vi "Conversion Lookup Table Get Conversion Parameter.vi"(8 "error in (no error)":errorcluster, 10 "ID":u32, 11 "Ref in":T2) -> (0 "error out":errorcluster {"code" min=0 max=0}, 1 "Found?":bool, 2 "Parameters":T1, 3 "vi reference":T2)   [LabVIEW 2013, in "J1939.lvlib"]
uses:
  J1939.lvlib
  LUTs/J1939 Conversion Lookup Table Reference.ctl
  LUTs/J1939 Conversion Lookup Table Parameters Cluster.ctl
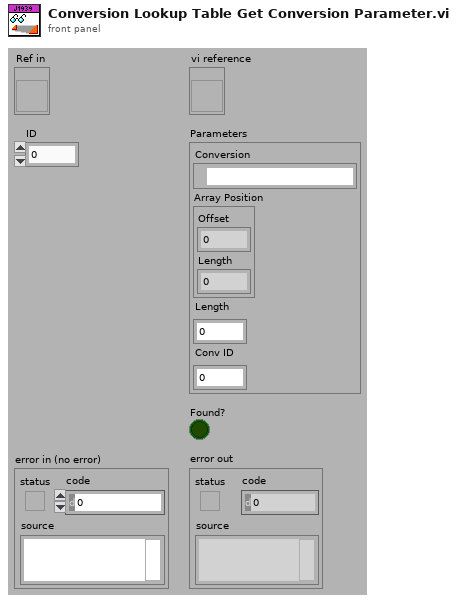
[diagram p1: front panel]
types:
  T1 = typedef "J1939.lvlib/J1939 Conversion Lookup Table Parameters Cluster.ctl" = cluster{"Conversion":refnum<k21>, "Array Position":cluster{"Offset":u32, "Length":u32}, "Length":u32, "Conv ID":u32}
  T2 = typedef "J1939.lvlib/J1939 Conversion Lookup Table Reference.ctl" = refnum<vi>
  T3 = typedef "J1939 Custom Device.lvlib/J1939 Conversion Lookup Table Parameters Cluster.ctl" = cluster{"Conversion":refnum<k21>, "Array Position":cluster{"Offset":u32, "Length":u32}, "Length":u32, "Conv ID":u32}
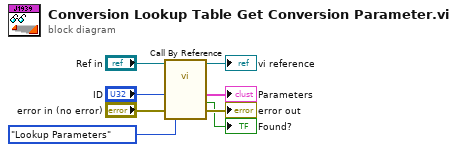
[diagram p0: block diagram]
diagram:
  n1 = call-by-ref "?"(reference="Ref in", "command"=enum16{"Set All", "Lookup Parameters"}."Lookup Parameters", "error in (no error)"="error in (no error)", "ID"="ID") -> (reference out=→"vi reference":T2, "error out"=→"error out":errorcluster, "Found?"=→"Found?":bool, "Parameters"=→"Parameters":T3)  [unwired: 7 in, 1 out]
